vi "CRYView Form Title Frame.vi"() -> ()   [LabVIEW 2013]
uses:
  <vilib>/Utility/miscctls.llb/LVPointTypeDef.ctl
  <vilib>/Utility/miscctls.llb/LVBoundsTypeDef.ctl
  <vilib>/Utility/miscctls.llb/LVPositionTypeDef.ctl
  SubVI/CRYMain Sub Window Global.vi
  CRYNew View Global.vi
  CRYCurveLibrary/Global/CRYCurve Library Global.vi
panel:
  in  "pSPRefParent":refnum<vi>
  in  "sClickState":string
  in  "nActiveState":i32
  in  "nIDFrame":i32
  in  "IconRing":u16(ring)
  in  "sViewName":string
  out "TitleName":string caption="Title Name"
  in  "StateOut":bool
  in  "stop":bool
  in  "InActiveClose":bool
  in  "ActiveClose":bool
  in  "bSPResize":bool
  in  "InActiveState":bool
  in  "ActiveStateHalf":bool
  out "SubVI Ref":refnum<vi>
  in  "ActiveState":bool
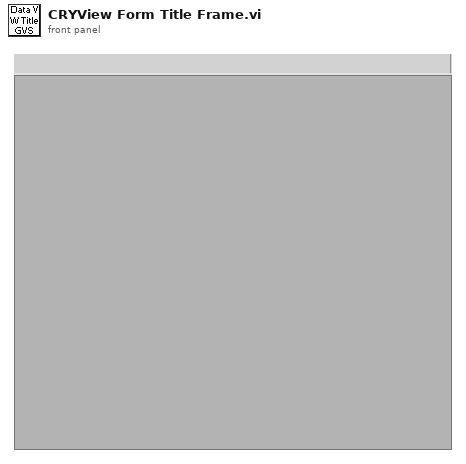
[diagram p1: front panel]
types:
  T1 = typedef "LVPointTypeDef.ctl" = cluster{"Horizontal":i16, "Vertical":i16}
  T2 = typedef "LVBoundsTypeDef.ctl" = cluster{"Width":u32, "Height":u32}
  T3 = typedef "LVPositionTypeDef.ctl" = cluster{"Left":i32, "Top":i32}
  T4 = typedef "LVRectTypeDef.ctl" = cluster{"Left":i16, "Top":i16, "Right":i16, "Bottom":i16}
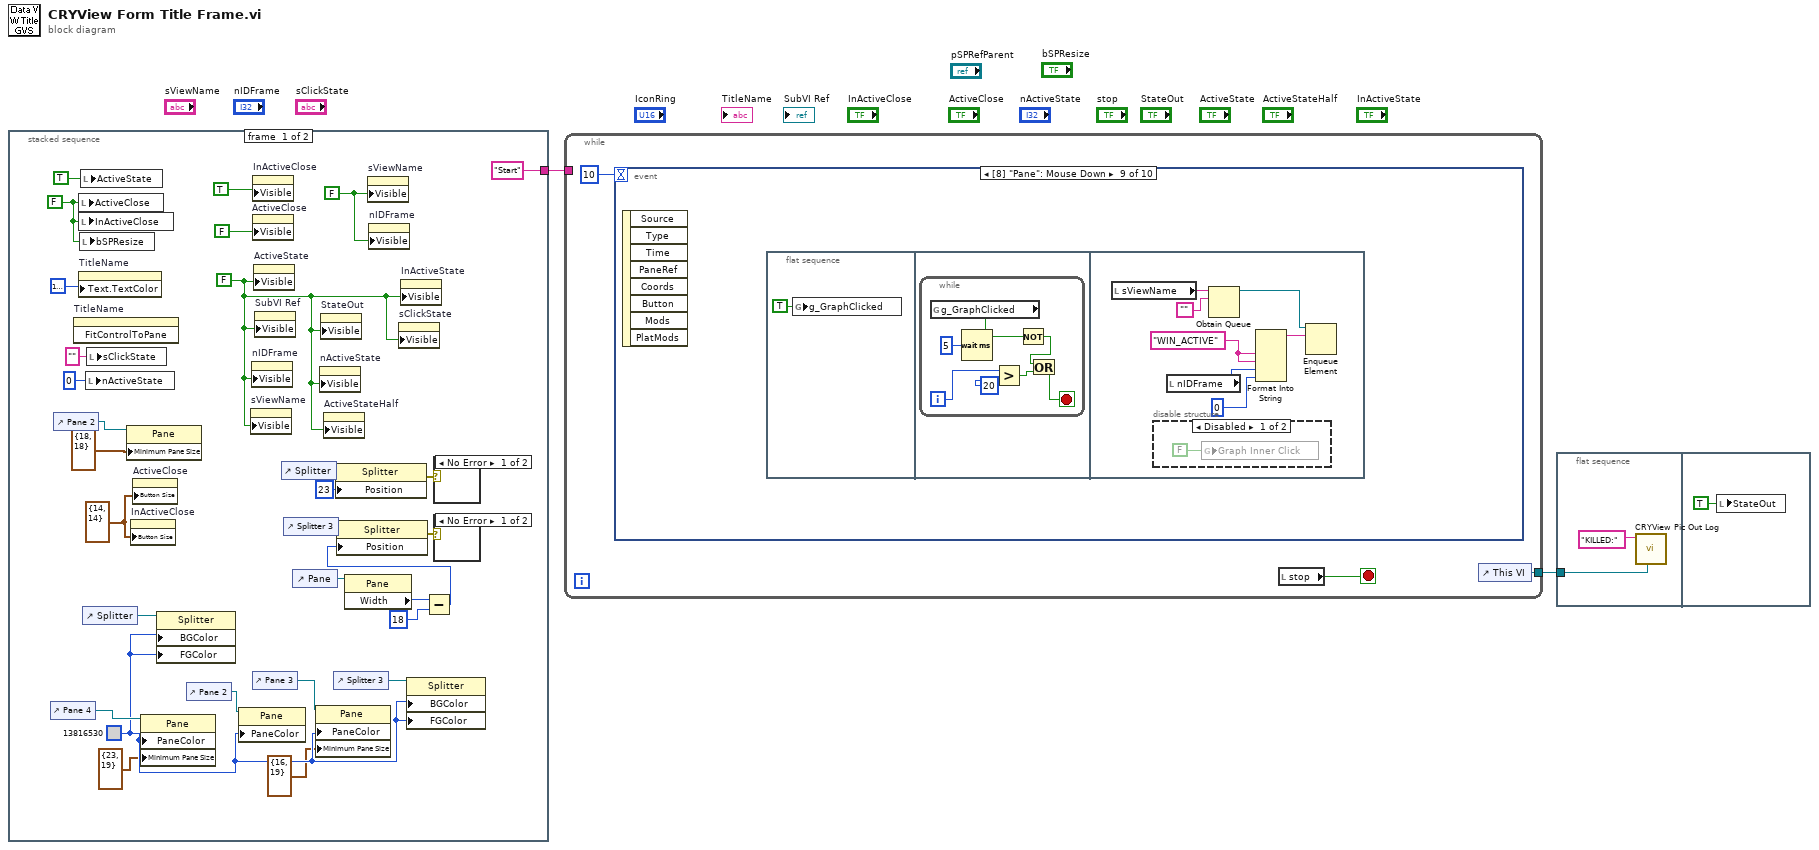
[diagram p0: block diagram]
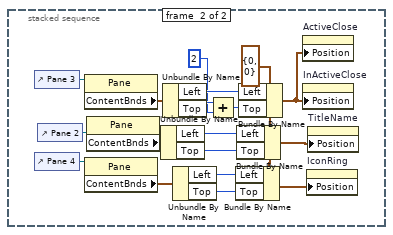
[diagram p4: hidden frame]
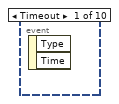
[diagram p5: hidden frame]
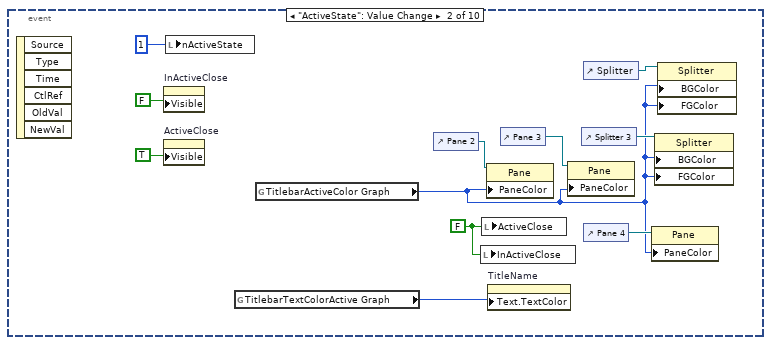
[diagram p6: hidden frame]
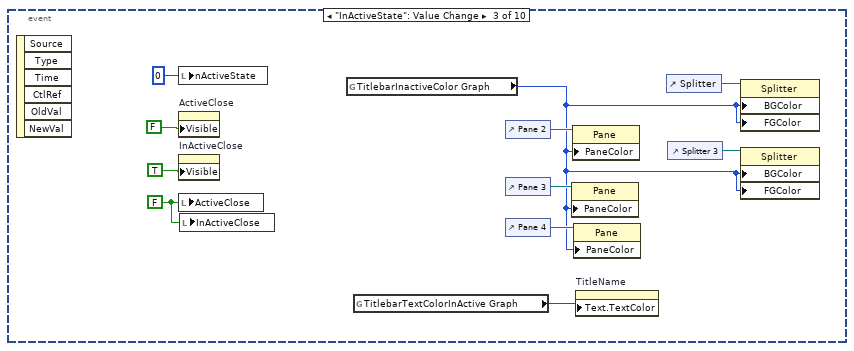
[diagram p7: hidden frame]
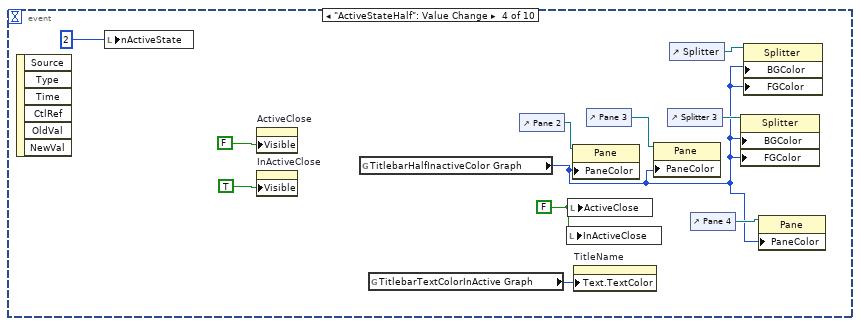
[diagram p8: hidden frame]
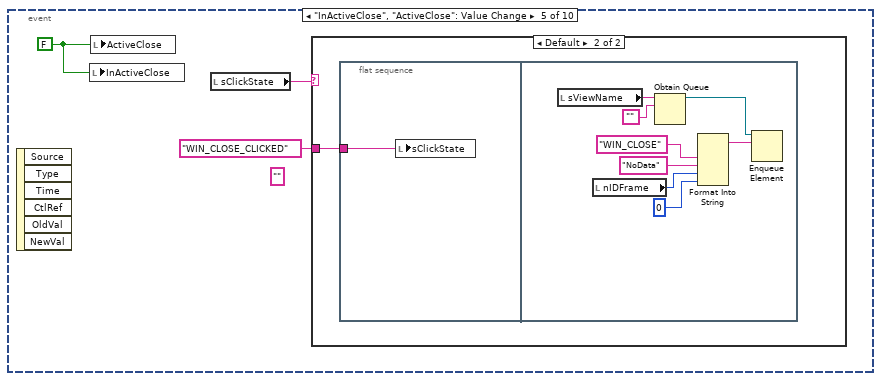
[diagram p9: hidden frame]
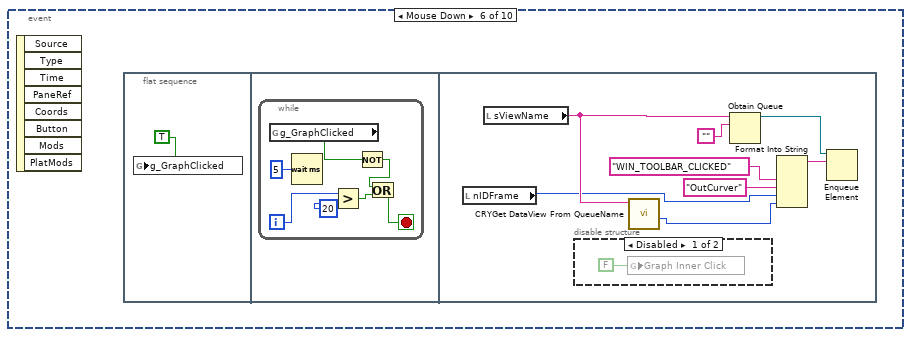
[diagram p11: hidden frame]
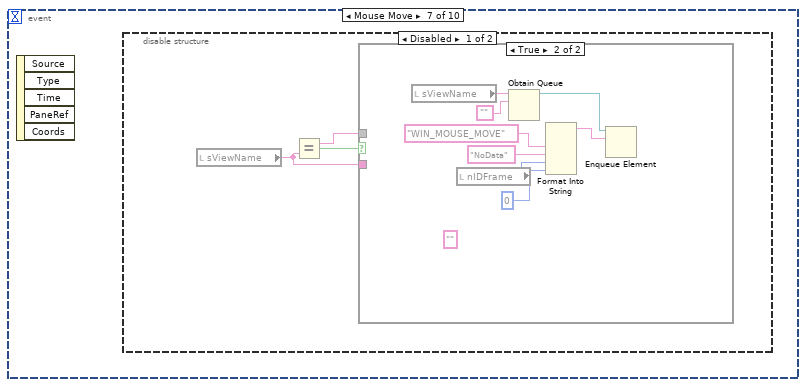
[diagram p13: hidden frame]
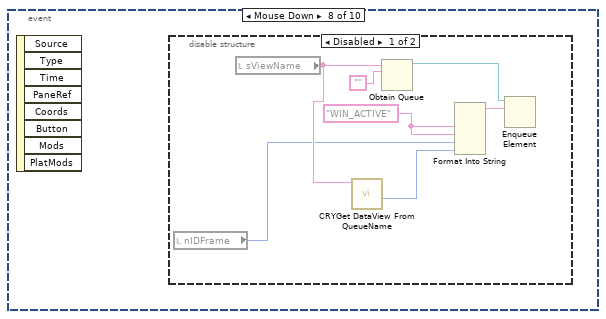
[diagram p16: hidden frame]
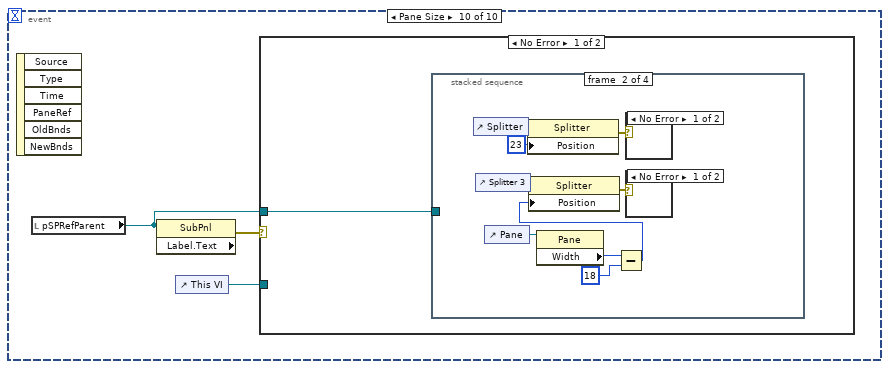
[diagram p19: hidden frame]
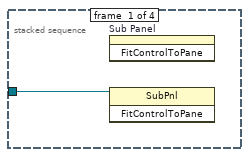
[diagram p20: hidden frame]
diagram:
  n1 = stacked-sequence {
    tunnel: ["Start" _] -> w1
    frame #0 {
      w19 = FALSE ("ToolBar Click")
      w21 = T2 {"Width"=14, "Height"=14} ("Button Size")
      w17 = FALSE ("ToolBar Click")
      w22 = u32 13816530
      w14 = FALSE ("Stop")
      n2 = control-ref of="Pane 4"() -> (w24:refnum<vi>)
      n3 = control-ref of="Pane 2"() -> (w26:refnum<vi>)
      n4 = invoke on="TitleName" class="Str" method="FitControlToPane"() -> ()  [unwired: 3 in, 3 out]
      n5 = local write "ActiveClose"(w14) -> ()
      n6 = local write "InActiveClose"(w14) -> ()
      n7 = property on="TitleName" class="Str"("Text.TextColor"=u32 16777222) -> ()  [unwired: 2 in, 2 out]
      n8 = local write "bSPResize"(w14) -> ()
      n9 = local write "ActiveState"(TRUE ("ActiveState")) -> ()
      n10 = control-ref of="Splitter"() -> (w23:refnum<vi>)
      n11 = local write "nActiveState"(0) -> ()
      n12 = local write "sClickState"("" ("sClickState")) -> ()
      n13 = property class="Pane"(reference=w26, "Minimum Pane Size"=T1 {"Horizontal"=18, "Vertical"=18}) -> ()  [unwired: 1 in, 2 out]
      n14 = property on="InActiveClose" class="Bool (strict)"("Button Size"=w21) -> ()  [unwired: 2 in, 2 out]
      n15 = property on="ActiveClose" class="Bool (strict)"("Button Size"=w21) -> ()  [unwired: 2 in, 2 out]
      n16 = property class="Pane"(reference=w24, "PaneColor"=w22, "Minimum Pane Size"=T1 {"Horizontal"=23, "Vertical"=19}) -> ()  [unwired: 1 in, 2 out]
      n17 = property class="Splitter"(reference=w23, "BGColor"=w22, "FGColor"=w22) -> ()  [unwired: 1 in, 2 out]
      n18 = control-ref of="Pane 2"() -> (w25:refnum<vi>)
      n19 = property class="Pane"(reference=w25, "PaneColor"=w22) -> ()  [unwired: 1 in, 2 out]
      n20 = property on="sViewName" class="Str"("Visible"=w17) -> ()  [unwired: 2 in, 2 out]
      n21 = property on="nIDFrame" class="DigNum (strict)"("Visible"=w17) -> ()  [unwired: 2 in, 2 out]
      n22 = property on="InActiveClose" class="Bool (strict)"("Visible"=TRUE ("ToolBar Click")) -> ()  [unwired: 2 in, 2 out]
      n23 = property on="ActiveClose" class="Bool (strict)"("Visible"=FALSE ("ToolBar Click")) -> ()  [unwired: 2 in, 2 out]
      n24 = control-ref of="Pane 3"() -> (w31:refnum<vi>)
      n25 = property on="ActiveState" class="Bool (strict)"("Visible"=w17) -> ()  [unwired: 2 in, 2 out]
      n26 = property on="SubVI Ref" class="VIRef (strict)"("Visible"=w17) -> ()  [unwired: 2 in, 2 out]
      n27 = control-ref of="Splitter"() -> (w5:refnum<vi>)
      n28 = control-ref of="Splitter 3"() -> (w6:refnum<vi>)
      n29 = control-ref of="Pane"() -> (w8:refnum<vi>)
      n30 = property class="Pane"(reference=w31, "PaneColor"=w22, "Minimum Pane Size"=T1 {"Horizontal"=16, "Vertical"=19}) -> ()  [unwired: 1 in, 2 out]
      n31 = property on="nActiveState" class="DigNum (strict)"("Visible"=w17) -> ()  [unwired: 2 in, 2 out]
      n32 = property on="StateOut" class="Bool (strict)"("Visible"=w17) -> ()  [unwired: 2 in, 2 out]
      n33 = property on="ActiveStateHalf" class="Bool (strict)"("Visible"=w17) -> ()  [unwired: 2 in, 2 out]
      n34 = control-ref of="Splitter 3"() -> (w30:refnum<vi>)
      n35 = property class="Splitter"(reference=w5, "Position"=23 ("Splitter Position")) -> (error out=w11:errorcluster)  [unwired: 1 in, 1 out]
      n36 = property class="Pane"(reference=w8) -> ("Width"=w9:u32)  [unwired: 1 in, 2 out]
      n37 = property on="sViewName" class="Str"("Visible"=w19) -> ()  [unwired: 2 in, 2 out]
      n38 = property on="nIDFrame" class="DigNum (strict)"("Visible"=w19) -> ()  [unwired: 2 in, 2 out]
      n39 = property on="sClickState" class="Str"("Visible"=w17) -> ()  [unwired: 2 in, 2 out]
      n40 = property on="InActiveState" class="Bool (strict)"("Visible"=w17) -> ()  [unwired: 2 in, 2 out]
      n41 = property class="Splitter"(reference=w30, "BGColor"=w22, "FGColor"=w22) -> ()  [unwired: 1 in, 2 out]
      n42 = Subtract(x=w9, y=u32 18) -> (x-y=w10:u32)
      n43 = property class="Splitter"(reference=w6, "Position"=w10) -> (error out=w12:errorcluster)  [unwired: 1 in, 1 out]
      n44 = case shown="No Error" w11 {
        frame No Error {
        }
        frame Error {
        }
      }
      n45 = case shown="No Error" w12 {
        frame No Error {
        }
        frame Error {
        }
      }
    }
    frame #1 {
      w50 = T3 {"Left"=0, "Top"=0} ("Position")
      n46 = control-ref of="Pane 3"() -> (w40:refnum<vi>)
      n47 = control-ref of="Pane 4"() -> (w48:refnum<vi>)
      n48 = control-ref of="Pane 2"() -> (w33:refnum<vi>)
      n49 = property class="Pane"(reference=w40) -> ("ContentBnds"=w39:T4)  [unwired: 1 in, 2 out]
      n50 = property class="Pane"(reference=w48) -> ("ContentBnds"=w46:T4)  [unwired: 1 in, 2 out]
      n51 = property class="Pane"(reference=w33) -> ("ContentBnds"=w43:T4)  [unwired: 1 in, 2 out]
      n52 = Unbundle By Name(w43) -> ("Left"=w42:i16, "Top"=w44:i16)
      n53 = Unbundle By Name(w39) -> ("Left"=w38:i16, "Top"=w36:i16)
      n54 = Unbundle By Name(w46) -> ("Left"=w47:i16, "Top"=w45:i16)
      n55 = Add(x=w36, y=i16 2) -> (x+y=w37:i16)
      n56 = Bundle By Name(cluster=w50, "Left"=w47, "Top"=w45) -> (w49:T3)
      n57 = Bundle By Name(cluster=w50, "Left"=w42, "Top"=w44) -> (w41:T3)
      n58 = Bundle By Name(cluster=w50, "Left"=w38, "Top"=w37) -> (w34:T3)
      n59 = property on="ActiveClose" class="Bool (strict)"("Position"=w34) -> ()  [unwired: 2 in, 2 out]
      n60 = property on="InActiveClose" class="Bool (strict)"("Position"=w34) -> ()  [unwired: 2 in, 2 out]
      n61 = property on="IconRing" class="Ring (strict)"("Position"=w49) -> ()  [unwired: 2 in, 2 out]
      n62 = property on="TitleName" class="Str"("Position"=w41) -> ()  [unwired: 2 in, 2 out]
    }
  }
  n63 = while {
    tunnel: [w52] -> w2
    tunnel: w1 -> [_]
    stop <- w51 stop-if-true
    n64 = event shown="[8] \"Pane\": Mouse Down" {
      selector: _ -> [_ _ _ _ _ _ _ _ _ _]
      dyn-events: _ -> [_ _ _ _ _ _ _ _ _ _]
      timeout: 10 -> [_ _ _ _ _ _ _ _ _ _]
      event Timeout {
        n65 = event-data() -> ()  [unwired: 3 out]
      }
      event "ActiveState": Value Change {
        w62 = FALSE ("Stop")
        n66 = event-data() -> ()  [unwired: 7 out]
        n67 = property on="InActiveClose" class="Bool (strict)"("Visible"=FALSE ("ToolBar Click")) -> ()  [unwired: 2 in, 2 out]
        n68 = property on="ActiveClose" class="Bool (strict)"("Visible"=TRUE ("ToolBar Click")) -> ()  [unwired: 2 in, 2 out]
        n69 = local write "nActiveState"(1) -> ()
        n70 = global read "CRYMain Sub Window Global.vi" "TitlebarTextColorActive Graph"() -> (w55:u32)
        n71 = global read "CRYMain Sub Window Global.vi" "TitlebarActiveColor Graph"() -> (w54:u32)
        n72 = control-ref of="Pane 2"() -> (w61:refnum<vi>)
        n73 = local write "InActiveClose"(w62) -> ()
        n74 = local write "ActiveClose"(w62) -> ()
        n75 = property class="Pane"(reference=w61, "PaneColor"=w54) -> ()  [unwired: 1 in, 2 out]
        n76 = property on="TitleName" class="Str"("Text.TextColor"=w55) -> ()  [unwired: 2 in, 2 out]
        n77 = control-ref of="Pane 3"() -> (w64:refnum<vi>)
        n78 = property class="Pane"(reference=w64, "PaneColor"=w54) -> ()  [unwired: 1 in, 2 out]
        n79 = control-ref of="Splitter 3"() -> (w63:refnum<vi>)
        n80 = control-ref of="Splitter"() -> (w59:refnum<vi>)
        n81 = control-ref of="Pane 4"() -> (w60:refnum<vi>)
        n82 = property class="Pane"(reference=w60, "PaneColor"=w54) -> ()  [unwired: 1 in, 2 out]
        n83 = property class="Splitter"(reference=w63, "BGColor"=w54, "FGColor"=w54) -> ()  [unwired: 1 in, 2 out]
        n84 = property class="Splitter"(reference=w59, "BGColor"=w54, "FGColor"=w54) -> ()  [unwired: 1 in, 2 out]
      }
      event "InActiveState": Value Change {
        w73 = FALSE ("Stop")
        n85 = event-data() -> ()  [unwired: 7 out]
        n86 = local write "nActiveState"(0) -> ()
        n87 = property on="ActiveClose" class="Bool (strict)"("Visible"=FALSE ("ToolBar Click")) -> ()  [unwired: 2 in, 2 out]
        n88 = property on="InActiveClose" class="Bool (strict)"("Visible"=TRUE ("ToolBar Click")) -> ()  [unwired: 2 in, 2 out]
        n89 = local write "ActiveClose"(w73) -> ()
        n90 = local write "InActiveClose"(w73) -> ()
        n91 = global read "CRYMain Sub Window Global.vi" "TitlebarInactiveColor Graph"() -> (w65:u32)
        n92 = global read "CRYMain Sub Window Global.vi" "TitlebarTextColorInActive Graph"() -> (w66:u32)
        n93 = control-ref of="Pane 2"() -> (w72:refnum<vi>)
        n94 = control-ref of="Pane 3"() -> (w75:refnum<vi>)
        n95 = control-ref of="Pane 4"() -> (w71:refnum<vi>)
        n96 = property class="Pane"(reference=w75, "PaneColor"=w65) -> ()  [unwired: 1 in, 2 out]
        n97 = property class="Pane"(reference=w72, "PaneColor"=w65) -> ()  [unwired: 1 in, 2 out]
        n98 = property class="Pane"(reference=w71, "PaneColor"=w65) -> ()  [unwired: 1 in, 2 out]
        n99 = property on="TitleName" class="Str"("Text.TextColor"=w66) -> ()  [unwired: 2 in, 2 out]
        n100 = control-ref of="Splitter"() -> (w70:refnum<vi>)
        n101 = control-ref of="Splitter 3"() -> (w74:refnum<vi>)
        n102 = property class="Splitter"(reference=w70, "BGColor"=w65, "FGColor"=w65) -> ()  [unwired: 1 in, 2 out]
        n103 = property class="Splitter"(reference=w74, "BGColor"=w65, "FGColor"=w65) -> ()  [unwired: 1 in, 2 out]
      }
      event "ActiveStateHalf": Value Change {
        w84 = FALSE ("Stop")
        n104 = event-data() -> ()  [unwired: 7 out]
        n105 = local write "nActiveState"(2) -> ()
        n106 = property on="ActiveClose" class="Bool (strict)"("Visible"=FALSE ("ToolBar Click")) -> ()  [unwired: 2 in, 2 out]
        n107 = property on="InActiveClose" class="Bool (strict)"("Visible"=TRUE ("ToolBar Click")) -> ()  [unwired: 2 in, 2 out]
        n108 = global read "CRYMain Sub Window Global.vi" "TitlebarHalfInactiveColor Graph"() -> (w77:u32)
        n109 = global read "CRYMain Sub Window Global.vi" "TitlebarTextColorInActive Graph"() -> (w76:u32)
        n110 = control-ref of="Pane 2"() -> (w83:refnum<vi>)
        n111 = local write "InActiveClose"(w84) -> ()
        n112 = local write "ActiveClose"(w84) -> ()
        n113 = property class="Pane"(reference=w83, "PaneColor"=w77) -> ()  [unwired: 1 in, 2 out]
        n114 = property on="TitleName" class="Str"("Text.TextColor"=w76) -> ()  [unwired: 2 in, 2 out]
        n115 = control-ref of="Pane 3"() -> (w86:refnum<vi>)
        n116 = property class="Pane"(reference=w86, "PaneColor"=w77) -> ()  [unwired: 1 in, 2 out]
        n117 = control-ref of="Splitter 3"() -> (w85:refnum<vi>)
        n118 = control-ref of="Splitter"() -> (w81:refnum<vi>)
        n119 = control-ref of="Pane 4"() -> (w82:refnum<vi>)
        n120 = property class="Splitter"(reference=w85, "BGColor"=w77, "FGColor"=w77) -> ()  [unwired: 1 in, 2 out]
        n121 = property class="Splitter"(reference=w81, "BGColor"=w77, "FGColor"=w77) -> ()  [unwired: 1 in, 2 out]
        n122 = property class="Pane"(reference=w82, "PaneColor"=w77) -> ()  [unwired: 1 in, 2 out]
      }
      event "InActiveClose", "ActiveClose": Value Change {
        w87 = FALSE ("Stop")
        (unwired) "" ("sData")
        n123 = event-data() -> ()  [unwired: 7 out]
        n124 = local write "InActiveClose"(w87) -> ()
        n125 = local write "ActiveClose"(w87) -> ()
        n126 = local read "sClickState"() -> (w89:string)
        n127 = case shown="Default" w89 {
          tunnel: "WIN_CLOSE_CLICKED" ("sData") -> [_ w90]
          frame "WIN_CLOSE_CLICKED" {
          }
          frame Default {
            n128 = flat-sequence {
              tunnel: w90 -> [w91]
              frame #0 {
                n129 = local write "sClickState"(w91) -> ()
              }
              frame #1 {
                n130 = local read "sViewName"() -> (w94:string)
                n131 = local read "nIDFrame"() -> (w96:i32)
                n132 = Obtain Queue(name (unnamed)=w94, element data type="") -> (queue out=w93:refnum<queue>)  [unwired: 3 in, 2 out]
                n133 = Format Into String("WIN_CLOSE" ("input 1"), "NoData" ("input 2"), w96, 0 ("input 3")) -> (resulting string=w92:string)  [unwired: 3 in, 1 out]
                n134 = Enqueue Element(queue=w93, element=w92) -> ()  [unwired: 1 in, 4 out]
              }
            }
          }
        }
      }
      event Mouse Down {
        n135 = event-data() -> ()  [unwired: 9 out]
        n136 = flat-sequence {
          frame #0 {
            n137 = global write "CRYNew View Global.vi" "g_GraphClicked"(TRUE ("g_GraphClicked")) -> ()
          }
          frame #1 {
            n138 = while {
              i -> [w106]
              stop <- w102 stop-if-true
              n139 = global read "CRYNew View Global.vi" "g_GraphClicked"() -> (w107:bool)
              n140 = Wait (ms)(milliseconds to wait=u32 5) -> ()  [unwired: 1 out]
              n141 = Greater?(x=w106, y=20) -> (0:w104:bool)
              n142 = Not(x=w107) -> (.not. x?=w103:bool)
              n143 = Or(x=w103, y=w104) -> (x .or. y?=w102:bool)
            }
          }
          frame #2 {
            n144 = local read "nIDFrame"() -> (w108:i32)
            n145 = local read "sViewName"() -> (w110:string)
            n146 = disable-structure shown="Disabled" {
              frame Disabled {
                n147 = global write "CRYCurve Library Global.vi" "Graph Inner Click"(FALSE ("Graph Inner Click")) -> ()
              }
              frame Enabled {
              }
            }
            n148 = call "CRYGet DataView From QueueName.vi"("DataView QueueName"=w110) -> ("DataView Idx out"=w109:i32)  [unwired: 8 in, 2 out]
            n149 = Obtain Queue(name (unnamed)=w110, element data type="") -> (queue out=w113:refnum<queue>)  [unwired: 3 in, 2 out]
            n150 = Format Into String("WIN_TOOLBAR_CLICKED" ("input 1"), "OutCurver" ("input 2"), w108, w109) -> (resulting string=w111:string)  [unwired: 3 in, 1 out]
            n151 = Enqueue Element(queue=w113, element=w111) -> ()  [unwired: 1 in, 4 out]
          }
        }
      }
      event Mouse Move {
        n152 = event-data() -> ()  [unwired: 6 out]
        n153 = disable-structure shown="Disabled" {
          frame Disabled {
            n154 = local read "sViewName"() -> (w117:string)
            n155 = Equal?(y=w117) -> (x=w118:string, x = y?=w119:bool)
            n156 = case shown="True" w119 {
              tunnel: w118 -> [_ _]
              tunnel: w117 -> [_ _]
              frame False {
              }
              frame True {
                w120 = "" ("sMouseMoveVIEWTitle")
                n157 = local read "sViewName"() -> (w122:string)
                n158 = local read "nIDFrame"() -> (w125:i32)
                n159 = Obtain Queue(name (unnamed)=w122, element data type="") -> (queue out=w124:refnum<queue>)  [unwired: 3 in, 2 out]
                n160 = Format Into String("WIN_MOUSE_MOVE" ("input 1"), "NoData" ("input 2"), w125, 0 ("input 3")) -> (resulting string=w121:string)  [unwired: 3 in, 1 out]
                n161 = Enqueue Element(queue=w124, element=w121) -> ()  [unwired: 1 in, 4 out]
              }
            }
          }
          frame Enabled {
          }
        }
      }
      event Mouse Down {
        n162 = event-data() -> ()  [unwired: 9 out]
        n163 = disable-structure shown="Disabled" {
          frame Disabled {
            w132 = "WIN_ACTIVE" ("input 1")
            n164 = local read "nIDFrame"() -> (w129:i32)
            n165 = local read "sViewName"() -> (w131:string)
            n166 = call "CRYGet DataView From QueueName.vi"("DataView QueueName"=w131) -> ("DataView Idx out"=w130:i32)  [unwired: 8 in, 2 out]
            n167 = Obtain Queue(name (unnamed)=w131, element data type="") -> (queue out=w135:refnum<queue>)  [unwired: 3 in, 2 out]
            n168 = Format Into String(w132, w132, w129, w130) -> (resulting string=w133:string)  [unwired: 3 in, 1 out]
            n169 = Enqueue Element(queue=w135, element=w133) -> ()  [unwired: 1 in, 4 out]
          }
          frame Enabled {
          }
        }
      }
      event Mouse Down {
        n170 = event-data() -> ()  [unwired: 9 out]
        n171 = flat-sequence {
          frame #0 {
            n172 = global write "CRYNew View Global.vi" "g_GraphClicked"(TRUE ("g_GraphClicked")) -> ()
          }
          frame #1 {
            n173 = while {
              i -> [w142]
              stop <- w138 stop-if-true
              n174 = global read "CRYNew View Global.vi" "g_GraphClicked"() -> (w143:bool)
              n175 = Wait (ms)(milliseconds to wait=u32 5) -> ()  [unwired: 1 out]
              n176 = Greater?(x=w142, y=20) -> (0:w140:bool)
              n177 = Not(x=w143) -> (.not. x?=w139:bool)
              n178 = Or(x=w139, y=w140) -> (x .or. y?=w138:bool)
            }
          }
          frame #2 {
            w144 = "WIN_ACTIVE" ("input 1")
            n179 = local read "sViewName"() -> (w146:string)
            n180 = disable-structure shown="Disabled" {
              frame Disabled {
                n181 = global write "CRYCurve Library Global.vi" "Graph Inner Click"(FALSE ("Graph Inner Click")) -> ()
              }
              frame Enabled {
              }
            }
            n182 = local read "nIDFrame"() -> (w149:i32)
            n183 = Obtain Queue(name (unnamed)=w146, element data type="") -> (queue out=w148:refnum<queue>)  [unwired: 3 in, 2 out]
            n184 = Format Into String(w144, w144, w149, 0 ("input 3")) -> (resulting string=w145:string)  [unwired: 3 in, 1 out]
            n185 = Enqueue Element(queue=w148, element=w145) -> ()  [unwired: 1 in, 4 out]
          }
        }
      }
      event Pane Size {
        n186 = event-data() -> ()  [unwired: 7 out]
        n187 = local read "pSPRefParent"() -> (w153:refnum<vi>)
        n188 = property class="SubPnl" props=["Label", "Text"](reference=w153) -> (error out=w154:errorcluster)  [unwired: 1 in, 2 out]
        n189 = control-ref of="This VI"() -> (w152:refnum<vi>)
        n190 = case shown="No Error" w154 {
          tunnel: w153 -> [w155 _]
          tunnel: w152 -> [_ _]
          frame No Error {
            n191 = stacked-sequence {
              tunnel: w155 -> [w156 _ _ _]
              frame #0 {
                n192 = invoke on="Sub Panel" class="SubPnl" method="FitControlToPane"() -> ()  [unwired: 3 in, 3 out]
                n193 = invoke class="SubPnl" method="FitControlToPane"(reference=w156) -> ()  [unwired: 2 in, 3 out]
              }
              frame #1 {
                n194 = control-ref of="Splitter"() -> (w157:refnum<vi>)
                n195 = control-ref of="Splitter 3"() -> (w158:refnum<vi>)
                n196 = control-ref of="Pane"() -> (w160:refnum<vi>)
                n197 = property class="Splitter"(reference=w157, "Position"=23 ("Splitter Position")) -> (error out=w163:errorcluster)  [unwired: 1 in, 1 out]
                n198 = property class="Pane"(reference=w160) -> ("Width"=w161:u32)  [unwired: 1 in, 2 out]
                n199 = Subtract(x=w161, y=u32 18) -> (x-y=w162:u32)
                n200 = property class="Splitter"(reference=w158, "Position"=w162) -> (error out=w164:errorcluster)  [unwired: 1 in, 1 out]
                n201 = case shown="No Error" w163 {
                  frame No Error {
                  }
                  frame Error {
                  }
                }
                n202 = case shown="No Error" w164 {
                  frame No Error {
                  }
                  frame Error {
                  }
                }
              }
              frame #2 {
                w166 = T3 {"Left"=0, "Top"=0} ("Position")
                n203 = control-ref of="Pane 3"() -> (w176:refnum<vi>)
                n204 = control-ref of="Pane 4"() -> (w168:refnum<vi>)
                n205 = control-ref of="Pane 2"() -> (w183:refnum<vi>)
                n206 = property class="Pane"(reference=w176) -> ("ContentBnds"=w177:T4)  [unwired: 1 in, 2 out]
                n207 = property class="Pane"(reference=w168) -> ("ContentBnds"=w170:T4)  [unwired: 1 in, 2 out]
                n208 = property class="Pane"(reference=w183) -> ("ContentBnds"=w173:T4)  [unwired: 1 in, 2 out]
                n209 = Unbundle By Name(w173) -> ("Left"=w174:i16, "Top"=w172:i16)
                n210 = Unbundle By Name(w177) -> ("Left"=w178:i16, "Top"=w180:i16)
                n211 = Unbundle By Name(w170) -> ("Left"=w169:i16, "Top"=w171:i16)
                n212 = Add(x=w180, y=i16 2) -> (x+y=w179:i16)
                n213 = Bundle By Name(cluster=w166, "Left"=w169, "Top"=w171) -> (w167:T3)
                n214 = Bundle By Name(cluster=w166, "Left"=w174, "Top"=w172) -> (w175:T3)
                n215 = Bundle By Name(cluster=w166, "Left"=w178, "Top"=w179) -> (w182:T3)
                n216 = property on="ActiveClose" class="Bool (strict)"("Position"=w182) -> ()  [unwired: 2 in, 2 out]
                n217 = property on="InActiveClose" class="Bool (strict)"("Position"=w182) -> ()  [unwired: 2 in, 2 out]
                n218 = property on="IconRing" class="Ring (strict)"("Position"=w167) -> ()  [unwired: 2 in, 2 out]
                n219 = property on="TitleName" class="Str"("Position"=w175) -> ()  [unwired: 2 in, 2 out]
              }
              frame #3 {
                n220 = local write "bSPResize"(TRUE ("bSPResize")) -> ()
              }
            }
          }
          frame Error {
            n221 = local write "bSPResize"(TRUE ("bSPResize")) -> ()
          }
        }
      }
    }
    n222 = local read "stop"() -> (w51:bool)
    n223 = control-ref of="This VI"() -> (w52:refnum<vi>)
  }
  n224 = flat-sequence {
    tunnel: w2 -> [w187]
    frame #0 {
      n225 = call "CRYView Pic Out Log.vi"("vi reference"=w187, "sData"="KILLED:") -> ()  [unwired: 10 in]
    }
    frame #1 {
      n226 = local write "StateOut"(TRUE ("StateOut")) -> ()
    }
  }
